vi "Set software shutter.vi"(8 "error in (no error)":errorcluster, 9 "Imaging Protocol":T1, 11 "Acquired z-plane index":i32) -> (0 "Error Out":errorcluster)   [LabVIEW 2017]
uses:
  Typedefs/Imaging Protocols enum.ctl
  Global Variables/gl_UI Ctrl Refs.vi
panel:
  out "Execution time (ms)":u32
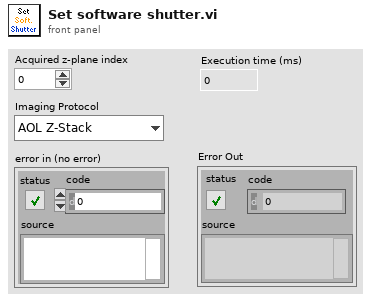
[diagram p1: front panel]
types:
  T1 = typedef "Imaging Protocols enum.ctl" = enum16{"AOL Z-Stack", "Motor Z Stack", "Functional Acquisition", "Single Plane Acquisition", "Volume Acquisition", "Live Imaging", "Live Plane Imaging", "Live Volume Imaging"}
  T2 = typedef "UI ctrl refs cluster.ctl" = cluster{"Top level VI path":path, "Top level VI ref":refnum<vi>, "User menu ref":refnum<k9>, "Sub Panel control":refnum<vi>, "Imaging Param Tab":refnum<vi>, "Occurrence-Start drivers":refnum<k4>, "Occurrence-Speed logging initialised":refnum<k4>, "Occurrence-XYZ stage initialised":refnum<k4>, "Exit button":refnum<vi>, "Status ind":refnum<vi>, "Set as origin":refnum<vi>, "Speed Logging":refnum<vi>, "Time Lapse":refnum<vi>, "Live Imaging":refnum<vi>, "AOL Z Stack":refnum<vi>, "Motor Z Stack":refnum<vi>, "Funct Acq button":refnum<vi>, "Hard Shutter":refnum<vi>, "Virtual Shutter":refnum<vi>, "Laser Power":refnum<vi>, "AOL Mode":refnum<vi>, "Frame Size":refnum<vi>, "Field of View":refnum<vi>, "Dwell Time":refnum<vi>, "Zoom":refnum<vi>, "AOL Z":refnum<vi>, "Objective":refnum<vi>, "Axis":refnum<vi>, "Paths & Names":refnum<vi>, "Experiment folder path (ind.)":refnum<vi>, "Last State (Ind.)":refnum<vi>, "Averages":refnum<vi>, "Angle (degrees)":refnum<vi>, "X centre":refnum<vi>, "Y centre":refnum<vi>, "Plane Mode":refnum<vi>, "# Planes":refnum<vi>, "Z Start":refnum<vi>, "Z Stop":refnum<vi>, "Z Step":refnum<vi>, "PMT 1":refnum<vi>, "PMT 2":refnum<vi>, "Stage XYZ Position":refnum<vi>, "Pockels@Z Start":refnum<vi>, "Pockels@Z Stop":refnum<vi>, "Obtain Z Start":refnum<vi>, "Obtain Z Stop":refnum<vi>, "Live stim.trig.period":refnum<vi>, "Live stim.trig.enable":refnum<vi>, "XY Stage Move":refnum<vi>, "Funct. Acq. Pockels Modulation":refnum<vi>, "Enable Video Recording":refnum<vi>, "Video Record-Live Imaging":refnum<vi>, "Video Record-Funct acq":refnum<vi>, "AOL Z-stack Chirps Ready (ind)":refnum<vi>, "Target time between mov.cor. ref triggers (ms)":refnum<vi>, "Center freq ind (nm)":refnum<vi>, "Pickup mode (ind)":refnum<vi>, "Logging queue (ind)":refnum<vi>, "Back aperture power (ind.)":refnum<vi>, "Power after objective (ind.)":refnum<vi>, "Switch user":refnum<vi>, "Ls1 Conn. Status":refnum<vi>, "Ls1Tuning Status":refnum<vi>, "Ls1 Faults":refnum<vi>, "Ls1 Connection":refnum<vi>, "Ls1 Mode":refnum<vi>, "Ls1 POWER [mW]":refnum<vi>, "Ls1Shutter":refnum<vi>, "Ls1 Wavelength":refnum<vi>, "Ls1 Note":refnum<vi>, "Ls1 Confirm Wav":refnum<vi>, "Ls1 PreChrp Prism1":refnum<vi>, "Ls1 PreChrp Prism2":refnum<vi>, "Ls1 wav top Ind":refnum<vi>, "Ls1 power top Ind":refnum<vi>, "Ls1 Pump peak Hold":refnum<vi>, "Ls1 Status Ind":refnum<vi>, "Ls1 wav cancel":refnum<vi>, "Experiment Type":refnum<vi>, "Biology Information":refnum<vi>}
  T3 = typedef "Laser control knob.ctl" = u16
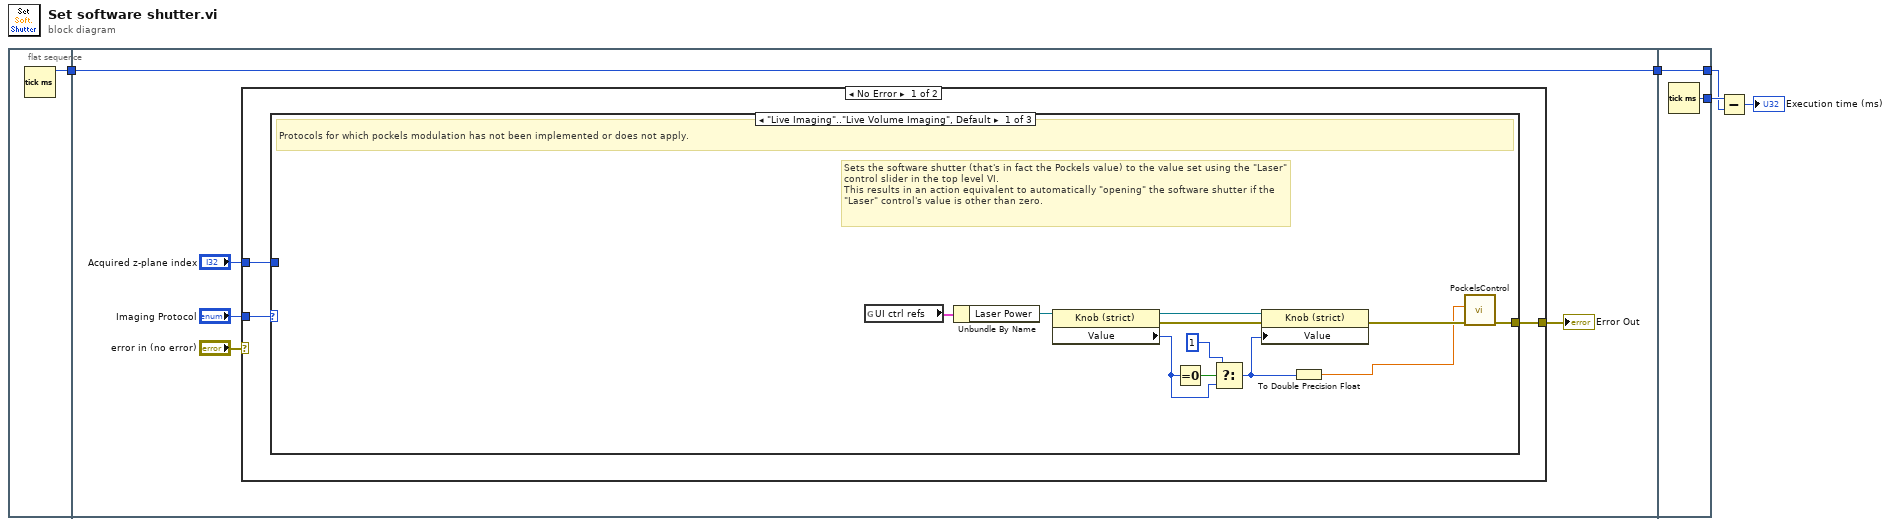
[diagram p0: block diagram]
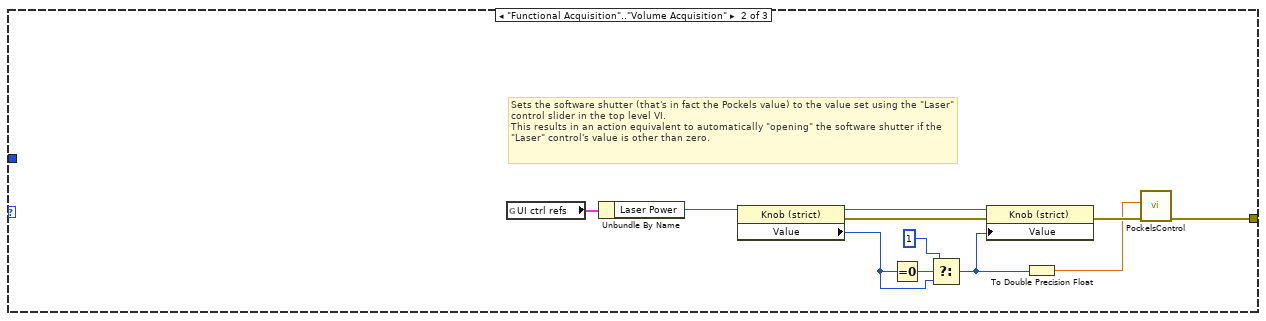
[diagram p2: hidden frame]
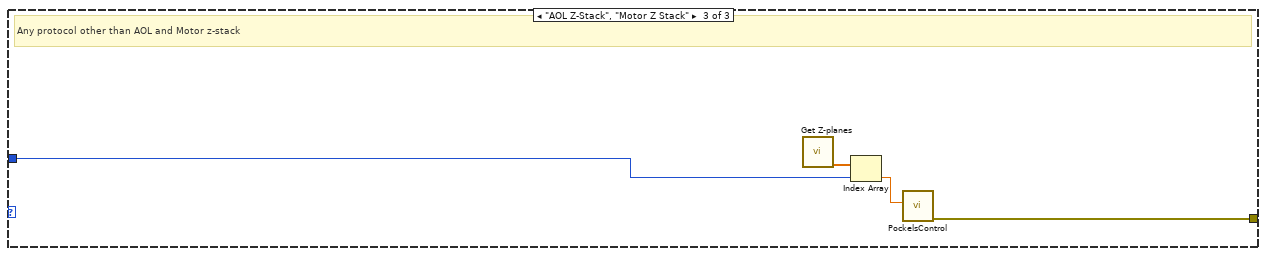
[diagram p3: hidden frame]
diagram:
  n1 = flat-sequence {
    tunnel: [w6] -> w4
    tunnel: w4 -> [w7]
    tunnel: [w7] -> w3
    tunnel: [w43] -> w5
    tunnel: w3 -> [w42]
    tunnel: [w42] -> w2
    frame #0 {
      n2 = Tick Count (ms)() -> (millisecond timer value=w6:u32)
    }
    frame #1 {
      n3 = case shown="No Error" "error in (no error)" {
        selector: "error in (no error)" -> [_ w41]
        tunnel: "Imaging Protocol" -> [w13 _]
        tunnel: "Acquired z-plane index" -> [w14 _]
        tunnel: [w12 w41] -> w8
        frame No Error {
          n4 = case shown="\"Live Imaging\"..\"Live Volume Imaging\", Default" w13 {
            tunnel: [w24 w26 w37] -> w12
            tunnel: w14 -> [_ _ w39]
            frame "Live Imaging".."Live Volume Imaging", Default {
              # "Sets the software shutter (that's in fact the Pockels value) to the value set using the \"Laser\" control slider in the top level VI. \nThis results in an action equivalent to automatically \"opening\" the software shutter if the \"Laser\" control's value is other than zero."
              # "Protocols for which pockels modulation has not been implemented or does not apply."
              n5 = global read "gl_UI Ctrl Refs.vi" "UI ctrl refs"() -> (w16:T2)
              n6 = Unbundle By Name(w16) -> ("Laser Power"=w15:refnum<vi>)
              n7 = property class="Knob (strict)"(reference=w15) -> (reference out=w19:refnum<vi>, error out=w18:errorcluster, "Value"=w20:T3)  [unwired: 1 in]
              n8 = Equal To 0?(x=w20) -> (x = 0?=w22:bool)
              n9 = Select(t=u16 1, s=w22, f=w20) -> (s? t:f=w17:T3)
              n10 = property class="Knob (strict)"(reference=w19, error in=w18, "Value"=w17) -> (error out=w25:errorcluster)  [unwired: 1 out]
              n11 = To Double Precision Float(number=w17) -> (double precision float=w23:dbl)
              n12 = call "PockelsControl.vi"("Error In"=w25, "Laser Power (%)"=w23) -> ("Error Out"=w24:errorcluster)  [unwired: 9 in]
            }
            frame "Functional Acquisition".."Volume Acquisition" {
              # "Sets the software shutter (that's in fact the Pockels value) to the value set using the \"Laser\" control slider in the top level VI. \nThis results in an action equivalent to automatically \"opening\" the software shutter if the \"Laser\" control's value is other than zero."
              n13 = global read "gl_UI Ctrl Refs.vi" "UI ctrl refs"() -> (w36:T2)
              n14 = Unbundle By Name(w36) -> ("Laser Power"=w35:refnum<vi>)
              n15 = property class="Knob (strict)"(reference=w35) -> (reference out=w31:refnum<vi>, error out=w30:errorcluster, "Value"=w32:T3)  [unwired: 1 in]
              n16 = Equal To 0?(x=w32) -> (x = 0?=w34:bool)
              n17 = Select(t=u16 1, s=w34, f=w32) -> (s? t:f=w29:T3)
              n18 = property class="Knob (strict)"(reference=w31, error in=w30, "Value"=w29) -> (error out=w28:errorcluster)  [unwired: 1 out]
              n19 = To Double Precision Float(number=w29) -> (double precision float=w27:dbl)
              n20 = call "PockelsControl.vi"("Error In"=w28, "Laser Power (%)"=w27) -> ("Error Out"=w26:errorcluster)  [unwired: 9 in]
            }
            frame "AOL Z-Stack", "Motor Z Stack" {
              # "Any protocol other than AOL and Motor z-stack"
              n21 = call "Get Z-planes.vi"() -> ("Pockels vs. Z (Laser power %)"=w40:dbl[])  [unwired: 7 in, 4 out]
              n22 = Index Array(array=w40, index=w39) -> (element=w38:dbl)
              n23 = call "PockelsControl.vi"("Laser Power (%)"=w38) -> ("Error Out"=w37:errorcluster)  [unwired: 10 in]
            }
          }
        }
        frame Error {
        }
      }
      "Error Out" <- w8
    }
    frame #2 {
      n24 = Tick Count (ms)() -> (millisecond timer value=w43:u32)
    }
  }
  n25 = Subtract(x=w5, y=w2) -> (x-y=→"Execution time (ms)":u32)
